vi "Labview görüntü işleme.vi"() -> ()   [LabVIEW 2018]
uses:
  <vilib>/userdefined/High Color/IMAQdx.ctl
  <vilib>/vision/driver/NI_Vision_Acquisition_Software.lvlib
panel:
  out "error out 3":errorcluster
  out "error out 2":errorcluster
  out "error out":errorcluster
  in  "Fotoğraf":bool
  out "Image":T1(plugin-control)
  in  "stop":bool
  in  "Session In":T2
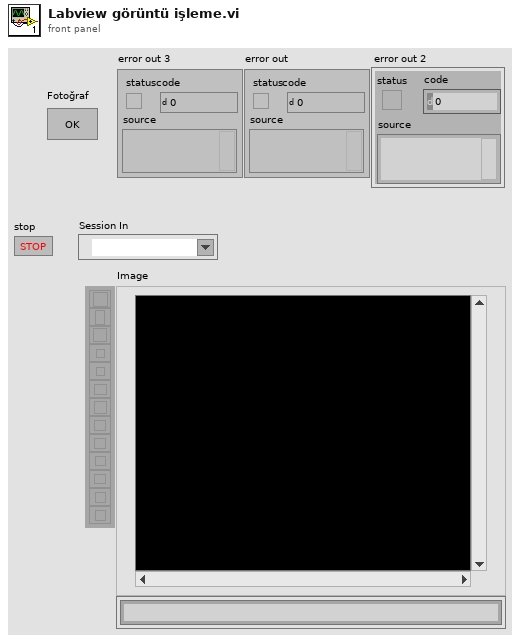
[diagram p1: front panel]
types:
  T1 = typedef "IMAQ Image.ctl" = refnum<image>
  T2 = typedef "IMAQdx.ctl" = refnum<k21>
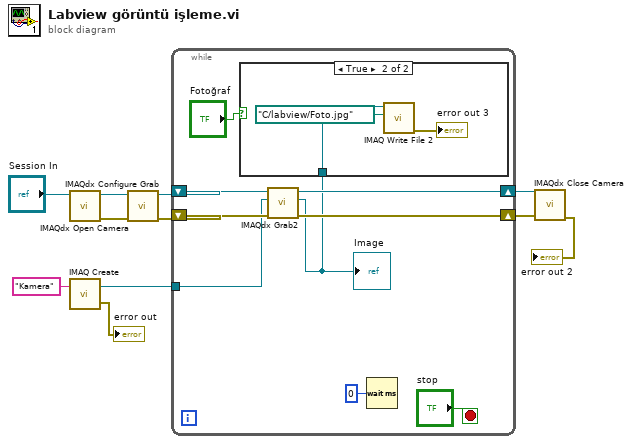
[diagram p0: block diagram]
diagram:
  n1 = call <vilib>:"IMAQdx Open Camera.vi"("Session In"="Session In") -> ("error out"=w7:errorcluster, "Session Out"=w10:T2)  [unwired: 9 in]
  n2 = call "IMAQ Create"("Image Name"="Kamera") -> ("New Image"=w3:T1, "error out"=→"error out":errorcluster)  [unwired: 4 in]
  n3 = call <vilib>:"IMAQdx Configure Grab.vi"("error in"=w7, "Session In"=w10) -> ("error out"=w6:errorcluster, "Session Out"=w9:T2)  [unwired: 8 in]
  n4 = while {
    tunnel: w3 -> [w16]
    shift-right: [w19] -> w8
    shift-left: w9 -> [w20]
    shift-right: [w17] -> w5
    shift-left: w6 -> [w18]
    stop <- "stop" stop-if-true
    n5 = call <vilib>:"IMAQdx Grab2.vi"("error in"=w18, "Image In"=w16, "Session In"=w20) -> ("error out"=w17:errorcluster, "Image Out"=w12:T1, "Session Out"=w19:T2)  [unwired: 5 in, 1 out]
    "Image" <- w12
    n6 = case shown="True" "Fotoğraf" {
      tunnel: w12 -> [_ w23]
      frame False {
      }
      frame True {
        n7 = call-poly "IMAQ Write File 2"("File Path"=path "C:/labview/Foto.jpg", "Image"=w23) -> ("error out"=→"error out 3":errorcluster)  [unwired: 8 in, 1 out]
      }
    }
    n8 = Wait (ms)(milliseconds to wait=u32 0) -> ()  [unwired: 1 out]
  }
  n9 = call <vilib>:"IMAQdx Close Camera.vi"("error in"=w5, "Session In"=w8) -> ("error out"=→"error out 2":errorcluster)  [unwired: 9 in]
